vi "UpdateRequestPersonnel.vi"(8 "error in":errorcluster, 9 "PersonnelType":enum16{"Dr", "Nurse"}(ring), 10 "RequestID":u32) -> (0 "error out":errorcluster)   [LabVIEW 2015, in "DatabaseApi.lvlib"]
uses:
  DatabaseApi.lvlib
  TypeDef/Request/RequestsTableColumnNamesRing.ctl
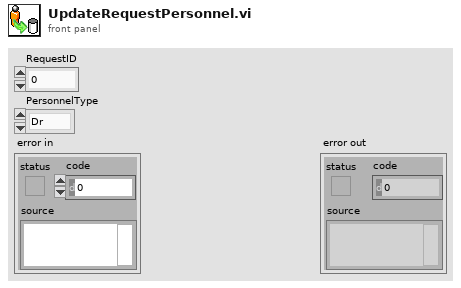
[diagram p1: front panel]
types:
  T1 = typedef "DatabaseApi.lvlib/RequestsTableColumnNamesRing.ctl" = enum16{"RequestID", "PersonnelType", "StartTime", "StartName", "AckTime", "AckName", "FulfilledTime", "FulfilledName", "Description"}
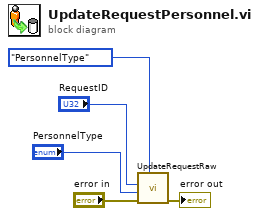
[diagram p0: block diagram]
diagram:
  n1 = call "UpdateRequestRaw.vi"("Data to update"=RequestsTableColumnNamesRing."PersonnelType", "error in"="error in", "data"="PersonnelType", "RequestID"="RequestID") -> ("error out"=→"error out":errorcluster)  [unwired: 7 in]
